vi "_builtins_align_selected.vi"(8 "error in (no error)":errorcluster, 9 "Align Type":T1, 10 "Panel":enum8{"FP", "BD"}(ring), 11 "VI Refnum in":refnum<vi>) -> (0 "error out":errorcluster, 3 "VI Refnum out":refnum<vi>)   [LabVIEW 2019, in "Script.lvlib"]
doc: "Aligns the selected front panel or block diagram objects excluding any display objects (i.e. labels, captions, inc/dec buttons, etc.)\n\nCreated by: Ryan Pacini"
uses:
  Script.lvlib
  _builtins_align.ctl
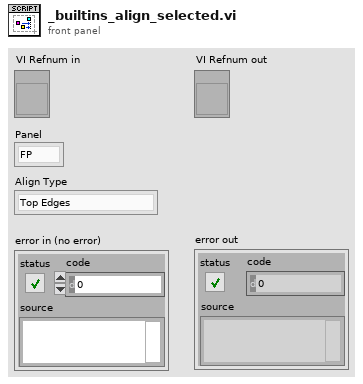
[diagram p1: front panel]
types:
  T1 = typedef "Script.lvlib/_builtins_align.ctl" = enum8{"Top Edges", "Vertical Centers", "Bottom Edges", "Left Edges", "Horizontal Centers", "Right Edges"}
  T2 = enum32{"Top Edges", "Vertical Centers", "Bottom Edges", "Left Edges", "Horizontal Centers", "Right Edges"}
  T3 = typedef "LVRectTypeDef.ctl" = cluster{"Left":i16, "Top":i16, "Right":i16, "Bottom":i16}
  T4 = typedef "LVPositionTypeDef.ctl" = cluster{"Left":i32, "Top":i32}
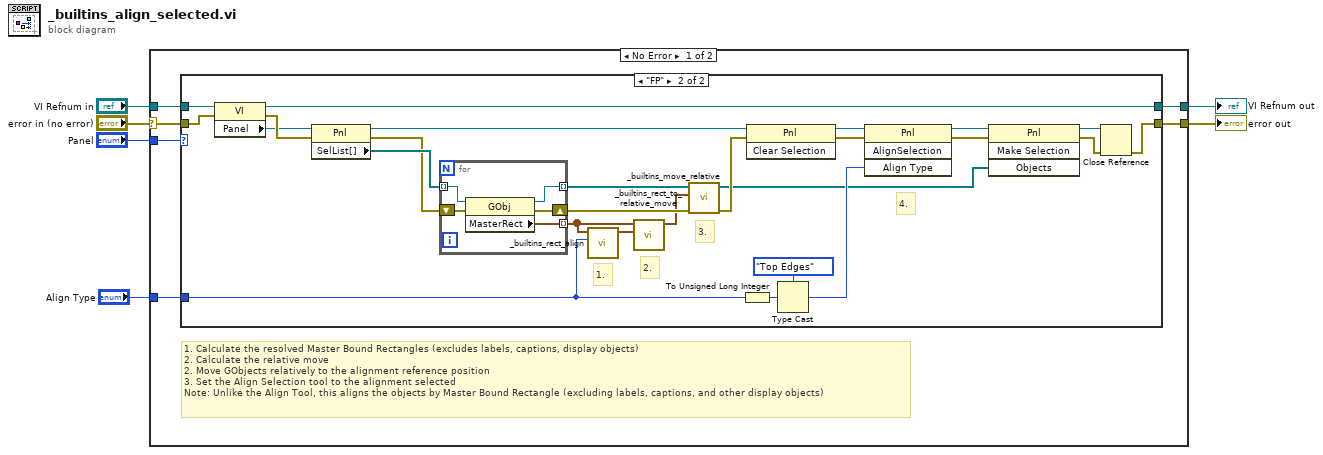
[diagram p0: block diagram]
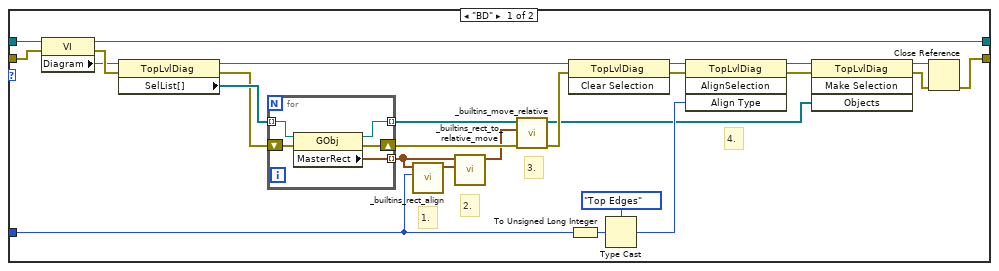
[diagram p2: hidden frame]
diagram:
  n1 = case shown="No Error" "error in (no error)" {
    selector: "error in (no error)" -> [w8 w75]
    tunnel: "Panel" -> [w12 _]
    tunnel: "VI Refnum in" -> [w11 w76]
    tunnel: [w10 w76] -> w4
    tunnel: [w9 w75] -> w3
    tunnel: "Align Type" -> [w7 _]
    frame No Error {
      # "1. Calculate the resolved Master Bound Rectangles (excludes labels, captions, display objects)\n2. Calculate the relative move\n2. Move GObjects relatively to the alignment reference position\n3. Set the Align Selection tool to the alignment selected\nNote: Unlike the Align Tool, this aligns the objects by Master Bound Rectangle (excluding labels, captions, and other display objects)"
      n2 = case shown="\"FP\"" w12 {
        tunnel: w8 -> [w37 w68]
        tunnel: w11 -> [w35 w66]
        tunnel: [w36 w67] -> w9
        tunnel: [w33 w64] -> w10
        tunnel: w7 -> [w25 w56]
        frame "BD" {
          # "2."
          # "3."
          # "4."
          # "1."
          n3 = property class="VI"(reference=w35, error in=w37) -> (reference out=w33:refnum<vi>, error out=w38:errorcluster, "Diagram"=w34:refnum<vi>)
          n4 = property class="TopLvlDiag"(reference=w34, error in=w38) -> (reference out=w32:refnum<vi>, error out=w18:errorcluster, "SelList[]"=w21:refnum<vi>[])
          n5 = for {
            tunnel: w21 -> [w43] mode=indexing
            tunnel: [w40] -> w14 mode=indexing
            shift-right: [w41] -> w16
            shift-left: w18 -> [w42]
            tunnel: [w39] -> w17 mode=indexing
            n6 = property class="GObj"(reference=w43, error in=w42) -> (reference out=w39:refnum<vi>, error out=w41:errorcluster, "MasterRect"=w40:T3)
          }
          n7 = call "_builtins_rect_align.vi"("Align Type"=w25, "Rects in"=w14) -> ("Resolved Rects out"=w15:T3[])  [unwired: 9 in]
          n8 = call "_builtins_rect_to_relative_move.vi"("End Rects out"=w15, "Start Rects in"=w14) -> ("Relative Move"=w13:T4[])  [unwired: 9 in]
          n9 = call "_builtins_move_relative.vi"("error in (no error)"=w16, "Relative Moves in"=w13, "GObjects in"=w17) -> ("error out"=w20:errorcluster, "GObjects out"=w19:refnum<vi>[])  [unwired: 7 in]
          n10 = invoke class="TopLvlDiag" method="Clear Selection"(reference=w32, error in=w20) -> (reference out=w28:refnum<vi>, error out=w27:errorcluster)  [unwired: 1 in, 1 out]
          n11 = To Unsigned Long Integer(number=w25) -> (unsigned 32bit integer=w26:u32)
          n12 = Type Cast(type=T2."Top Edges" ("Align Type"), x=w26) -> (*(type *) &x=w24:T2)
          n13 = invoke class="TopLvlDiag" method="AlignSelection"(reference=w28, error in=w27, "Align Type"=w24) -> (reference out=w31:refnum<vi>, error out=w29:errorcluster)  [unwired: 1 in, 2 out]
          n14 = invoke class="TopLvlDiag" method="Make Selection"(reference=w31, error in=w29, "Objects"=w19) -> (reference out=w30:refnum<vi>, error out=w23:errorcluster)  [unwired: 1 in, 2 out]
          n15 = Close Reference(reference=w30, error in (no error)=w23) -> (error out=w36:errorcluster)
        }
        frame "FP" {
          # "3."
          # "2."
          # "4."
          # "1."
          n16 = property class="VI"(reference=w66, error in=w68) -> (reference out=w64:refnum<vi>, error out=w69:errorcluster, "Panel"=w65:refnum<vi>)
          n17 = property class="Pnl"(reference=w65, error in=w69) -> (reference out=w63:refnum<vi>, error out=w49:errorcluster, "SelList[]"=w52:refnum<vi>[])
          n18 = for {
            tunnel: w52 -> [w74] mode=indexing
            tunnel: [w71] -> w46 mode=indexing
            shift-right: [w72] -> w47
            shift-left: w49 -> [w73]
            tunnel: [w70] -> w48 mode=indexing
            n19 = property class="GObj"(reference=w74, error in=w73) -> (reference out=w70:refnum<vi>, error out=w72:errorcluster, "MasterRect"=w71:T3)
          }
          n20 = call "_builtins_rect_align.vi"("Align Type"=w56, "Rects in"=w46) -> ("Resolved Rects out"=w45:T3[])  [unwired: 9 in]
          n21 = call "_builtins_rect_to_relative_move.vi"("End Rects out"=w45, "Start Rects in"=w46) -> ("Relative Move"=w44:T4[])  [unwired: 9 in]
          n22 = call "_builtins_move_relative.vi"("error in (no error)"=w47, "Relative Moves in"=w44, "GObjects in"=w48) -> ("error out"=w51:errorcluster, "GObjects out"=w50:refnum<vi>[])  [unwired: 7 in]
          n23 = To Unsigned Long Integer(number=w56) -> (unsigned 32bit integer=w57:u32)
          n24 = invoke class="Pnl" method="Clear Selection"(reference=w63, error in=w51) -> (reference out=w59:refnum<vi>, error out=w58:errorcluster)  [unwired: 1 in, 1 out]
          n25 = Type Cast(type=T2."Top Edges" ("Align Type"), x=w57) -> (*(type *) &x=w55:T2)
          n26 = invoke class="Pnl" method="AlignSelection"(reference=w59, error in=w58, "Align Type"=w55) -> (reference out=w62:refnum<vi>, error out=w60:errorcluster)  [unwired: 1 in, 2 out]
          n27 = invoke class="Pnl" method="Make Selection"(reference=w62, error in=w60, "Objects"=w50) -> (reference out=w61:refnum<vi>, error out=w54:errorcluster)  [unwired: 1 in, 2 out]
          n28 = Close Reference(reference=w61, error in (no error)=w54) -> (error out=w67:errorcluster)
        }
      }
    }
    frame Error {
    }
  }
  "VI Refnum out" <- w4
  "error out" <- w3
